vi "Launch Dialog Box.vi"(8 "error in (no error)":errorcluster, 10 "DialogBox":refnum<class "IDialogBox.lvclass">, 11 "DialogBoxViewable in":refnum<class "DialogBoxViewManager.lvclass">) -> (0 "error out":errorcluster, 3 "DialogBoxViewable out":refnum<class "DialogBoxViewManager.lvclass">)   [LabVIEW 2019, in "DialogBoxViewManager.lvlib" / "DialogBoxViewManager.lvclass"]
uses:
  <vilib>/gpm_packages/@cs/mva-dialogbox/source/DialogBoxViewManager/DialogBoxViewManager/DialogBoxViewManager.lvclass
  C:/Program Files/National Instruments/LabVIEW 2019/vi.lib/ActorFramework/Actor/Actor.lvclass
  C:/Program Files/National Instruments/LabVIEW 2019/vi.lib/gpm_packages/@cs/mva-viewable/Source/IViewable/IViewable/IViewable.lvclass
  <vilib>/gpm_packages/@cs/mva-dialogbox/source/IDialogBox/IDialogBox/IDialogBox.lvclass
  <vilib>/gpm_packages/@cs/mva-dialogbox/source/DialogBoxViewManager/DialogBoxViewManager/DialogBoxViewManager.lvclass/DialogBoxViewManager.ctl
  <vilib>/gpm_packages/@cs/mva-viewable/Source/IViewable/IViewable/IViewable.lvclass/IViewable.ctl
  <vilib>/gpm_packages/@cs/mva-core/Source/IObserver/IObserver/IObserver.lvclass/IObserver.ctl
  <vilib>/ActorFramework/Message Enqueuer/Message Enqueuer.lvclass/Message Enqueuer.ctl
  <vilib>/ActorFramework/Message Enqueuer/Enqueue.vi
  <vilib>/gpm_packages/@cs/mva-viewable/Source/IViewable/IViewable/Write Application Style Reference.vi
  <vilib>/gpm_packages/@cs/mva-viewable/Source/IViewable/IViewable/Read Application Style Reference.vi
  <vilib>/gpm_packages/@cs/mva-core/Source/IObserver/IObserver/Transfer Observer Resources.vi
  <vilib>/gpm_packages/@cs/mva-viewable/Source/IViewable/IViewable/IViewable.lvclass
  C:/Program Files/National Instruments/LabVIEW 2019/vi.lib/gpm_packages/@cs/mva-core/Source/IObserver/IObserver/IObserver.lvclass
  <vilib>/ActorFramework/Stop Msg/Stop Msg.lvclass
  C:/Program Files/National Instruments/LabVIEW 2019/vi.lib/ActorFramework/Message/Message.lvclass
  <vilib>/ActorFramework/Message Priority Queue/Priority Enqueue.vi
  <vilib>/ActorFramework/Actor/Actor.lvclass
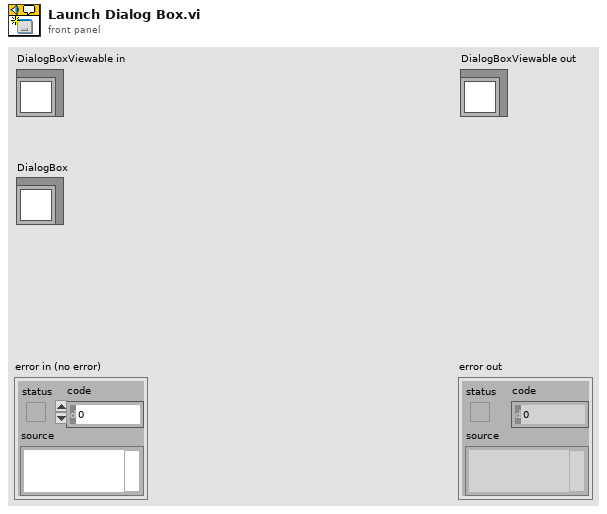
[diagram p1: front panel]
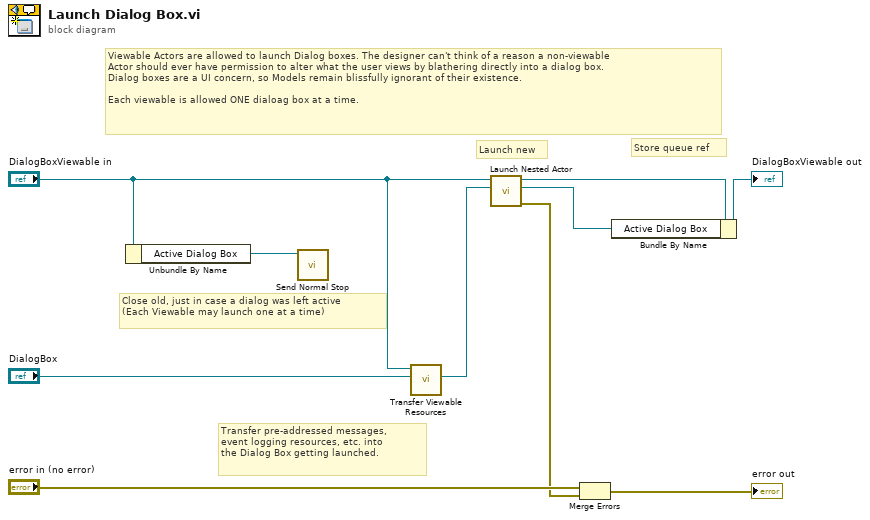
[diagram p0: block diagram]
diagram:
  # "Transfer pre-addressed messages,\nevent logging resources, etc. into\nthe Dialog Box getting launched."
  # "Store queue ref"
  # "Launch new"
  # "Viewable Actors are allowed to launch Dialog boxes. The designer can't think of a reason a non-viewable\nActor should ever have permission to alter what the user views by blathering directly into a dialog box.\nDialog boxes are a UI concern, so Models remain blissfully ignorant of their existence.\n\nEach viewable is allowed ONE dialoag box at a time."
  # "Close old, just in case a dialog was left active\n(Each Viewable may launch one at a time)"
  n1 = Unbundle By Name("DialogBoxViewable in") -> ("Active Dialog Box"=w9:refnum<class "Message Enqueuer.lvclass">)
  n2 = call <vilib>:"Send Normal Stop.vi"("Message Enqueuer"=w9) -> ()  [unwired: 10 in, 1 out]
  n3 = call <vilib>:"Transfer Viewable Resources.vi"("Recipient Viewable In"="DialogBox", "Running Viewable"="DialogBoxViewable in") -> ("Recipient Viewable Out"=w1:refnum<class "IDialogBox.lvclass">)  [unwired: 9 in]
  n4 = call <vilib>:"Launch Nested Actor.vi"("Nested Actor"=w1, "Caller Actor in"="DialogBoxViewable in") -> ("error out"=w4:errorcluster, "Nested Actor's Enqueuer"=w6:refnum<class "Message Enqueuer.lvclass">, "Caller Actor out"=w8:refnum<class "DialogBoxViewManager.lvclass">)  [unwired: 7 in]
  n5 = Merge Errors("error in (no error)", w4) -> (→"error out":errorcluster)
  n6 = Bundle By Name(cluster=w8, "Active Dialog Box"=w6) -> (→"DialogBoxViewable out":refnum<class "DialogBoxViewManager.lvclass">)
